vi "continue file.vi"(4 "sampling rate":dbl, 5 "accel range":dbl, 6 "counts per rev":dbl, 7 "gyro range":dbl, 8 "error in (no error)":errorcluster, 10 "original file":refnum<k34>, 11 "original path":path) -> (0 "error out":errorcluster, 1 "channel names":string[](array[string]), 2 "tdms file out":refnum<k34>, 3 "incremented path":path)   [LabVIEW 2012]
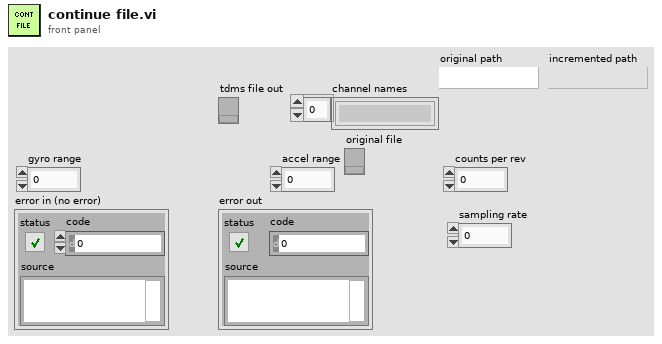
[diagram p1: front panel]
types:
  T1 = enum16{"open", "open or create", "create or replace", "create", "open (read-only)"}
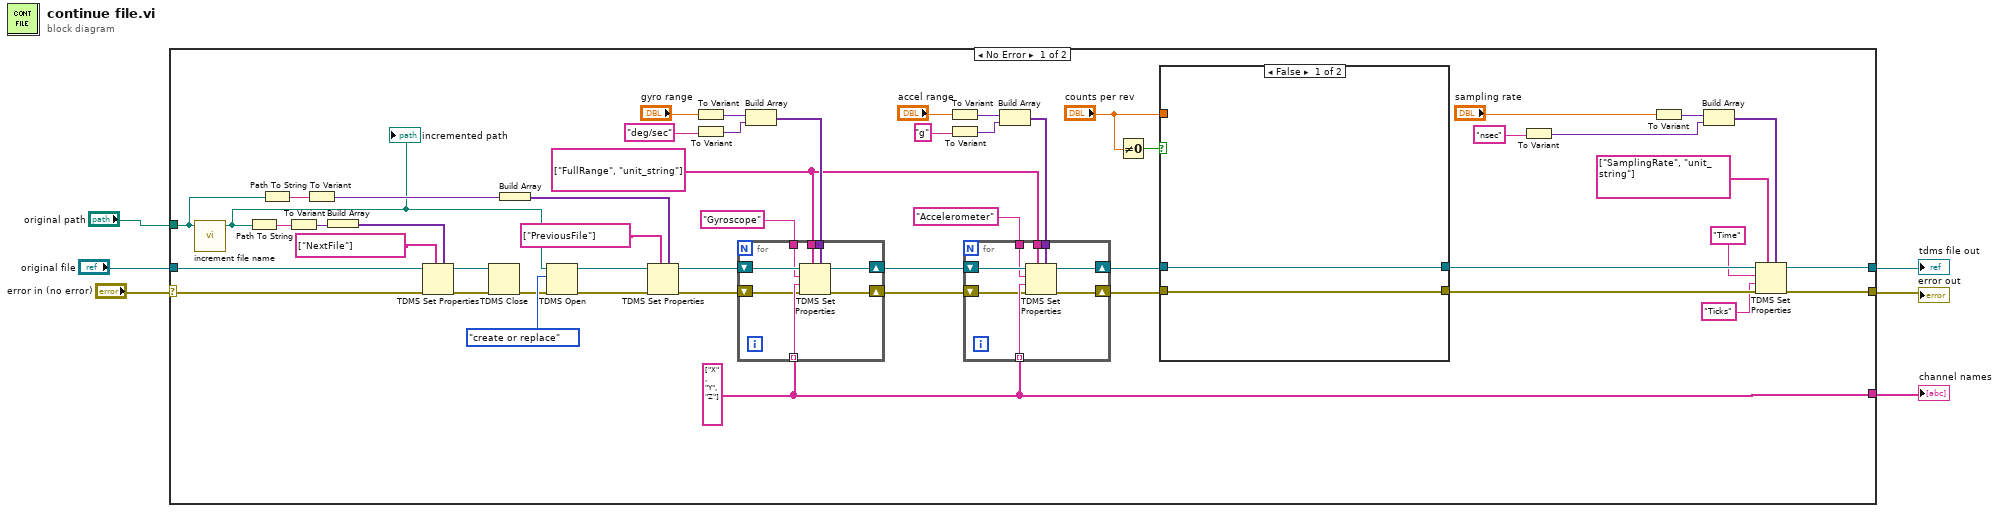
[diagram p0: block diagram]
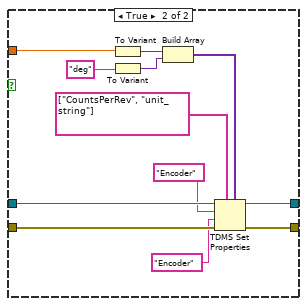
[diagram p2: hidden frame]
diagram:
  n1 = case shown="No Error" "error in (no error)" {
    selector: "error in (no error)" -> [w21 w89]
    tunnel: "original file" -> [w25 _]
    tunnel: [w34 _] -> w5
    tunnel: [w33 w89] -> w4
    tunnel: [w42 _] -> w3
    tunnel: "original path" -> [w16 _]
    frame No Error {
      w48 = string[] ["FullRange", "unit_string"] ("property names")
      w42 = string[] ["X", "Y", "Z"] ("channel name(s)")
      n2 = call "increment file name.vi"("file path in"=w16) -> ("incremented path"=w9:path)  [unwired: 10 in]
      "incremented path" <- w9
      n3 = Path To String(path=w9) -> (string=w7:string)
      n4 = Path To String(path=w16) -> (string=w8:string)
      n5 = To Variant(anything=w7) -> (Variant=w23:variant)
      n6 = To Variant(anything=w8) -> (Variant=w15:variant)
      n7 = Build Array(w23) -> (w22:variant[])
      n8 = TDMS Set Properties(5:w22, 7:string[] ["NextFile"] ("property names"), 8:w21, 11:w25) -> (0:w19:errorcluster, 3:w20:refnum<k34>)  [unwired: 2 in, 2 out]
      n9 = TDMS Close(8:w19, 11:w20) -> (0:w10:errorcluster)  [unwired: 1 out]
      n10 = Build Array(w15) -> (w18:variant[])
      n11 = TDMS Open(8:w10, 10:T1."create or replace" ("operation (0:open)"), 11:w9) -> (0:w13:errorcluster, 3:w14:refnum<k34>)  [unwired: 3 in]
      n12 = TDMS Set Properties(5:w18, 7:string[] ["PreviousFile"] ("property names"), 8:w13, 11:w14) -> (0:w11:errorcluster, 3:w12:refnum<k34>)  [unwired: 2 in, 2 out]
      n13 = To Variant(anything="gyro range") -> (Variant=w54:variant)
      n14 = To Variant(anything="deg/sec" ("group name (Untitled)")) -> (Variant=w53:variant)
      n15 = Build Array(w54, w53) -> (w52:variant[])
      n16 = for {
        tunnel: "Gyroscope" ("group name (Untitled)") -> [w87]
        tunnel: w42 -> [w86] mode=indexing
        shift-right: [w84] -> w49
        shift-left: w11 -> [w85]
        tunnel: w48 -> [w83]
        tunnel: w52 -> [w82]
        shift-right: [w81] -> w50
        shift-left: w12 -> [w88]
        n17 = TDMS Set Properties(5:w82, 7:w83, 8:w85, 9:w86, 10:w87, 11:w88) -> (0:w84:errorcluster, 3:w81:refnum<k34>)  [unwired: 2 out]
      }
      n18 = To Variant(anything="accel range") -> (Variant=w46:variant)
      n19 = To Variant(anything="g" ("group name (Untitled)")) -> (Variant=w47:variant)
      n20 = Build Array(w46, w47) -> (w43:variant[])
      n21 = for {
        tunnel: "Accelerometer" ("group name (Untitled)") -> [w79]
        tunnel: w42 -> [w78] mode=indexing
        shift-right: [w76] -> w40
        shift-left: w49 -> [w77]
        tunnel: w48 -> [w75]
        tunnel: w43 -> [w74]
        shift-right: [w73] -> w41
        shift-left: w50 -> [w80]
        n22 = TDMS Set Properties(5:w74, 7:w75, 8:w77, 9:w78, 10:w79, 11:w80) -> (0:w76:errorcluster, 3:w73:refnum<k34>)  [unwired: 2 out]
      }
      n23 = Not Equal To 0?(x="counts per rev") -> (x != 0?=w38:bool)
      n24 = case shown="False" w38 {
        tunnel: w41 -> [w60 w72]
        tunnel: [w60 w71] -> w36
        tunnel: w40 -> [w59 w70]
        tunnel: [w59 w69] -> w35
        tunnel: "counts per rev" -> [_ w68]
        frame False {
        }
        frame True {
          n25 = To Variant(anything=w68) -> (Variant=w66:variant)
          n26 = To Variant(anything="deg" ("group name (Untitled)")) -> (Variant=w65:variant)
          n27 = Build Array(w66, w65) -> (w64:variant[])
          n28 = TDMS Set Properties(5:w64, 7:string[] ["CountsPerRev", "unit_string"] ("property names"), 8:w70, 9:"Encoder" ("group name"), 10:"Encoder" ("group name"), 11:w72) -> (0:w69:errorcluster, 3:w71:refnum<k34>)  [unwired: 2 out]
        }
      }
      n29 = To Variant(anything="nsec" ("group name (Untitled)")) -> (Variant=w26:variant)
      n30 = To Variant(anything="sampling rate") -> (Variant=w32:variant)
      n31 = Build Array(w32, w26) -> (w31:variant[])
      n32 = TDMS Set Properties(5:w31, 7:string[] ["SamplingRate", "unit_string"] ("property names"), 8:w35, 9:"Ticks" ("group name"), 10:"Time" ("group name"), 11:w36) -> (0:w33:errorcluster, 3:w34:refnum<k34>)  [unwired: 2 out]
    }
    frame Error {
    }
  }
  "tdms file out" <- w5
  "error out" <- w4
  "channel names" <- w3
